vi "DSF.Engine.Timing.Max Concurrent Activations.vi"(8 "error in (no error)":errorcluster, 11 "Timings in":refnum<class "DSF.Engine.Timing.lvclass">[](array[class])) -> (0 "error out":errorcluster, 3 "Timings out":refnum<class "DSF.Engine.Timing.lvclass">[](array[class]))   [LabVIEW 2017, in "DSF.Engine.lvlib" / "DSF.Engine.Timing.lvclass"]
uses:
  DSF.Engine.Timing.lvclass
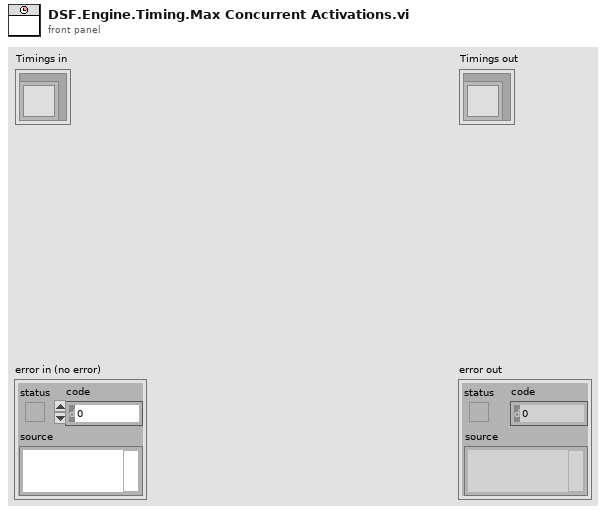
[diagram p1: front panel]
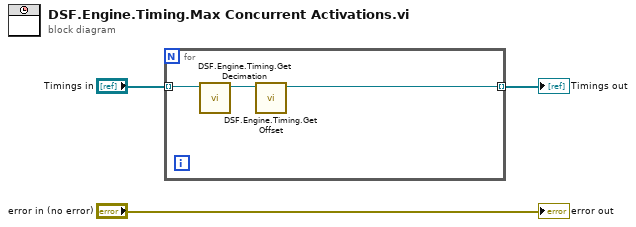
[diagram p0: block diagram]
diagram:
  n1 = for {
    tunnel: "Timings in" -> [w6] mode=indexing
    tunnel: [w4] -> w1 mode=indexing
    n2 = call "DSF.Engine.Timing.Get Decimation.vi"("Timing in"=w6) -> ("Timing out"=w5:refnum<class "DSF.Engine.Timing.lvclass">)  [unwired: 9 in, 1 out]
    n3 = call "DSF.Engine.Timing.Get Offset.vi"("Timing in"=w5) -> ("Timing out"=w4:refnum<class "DSF.Engine.Timing.lvclass">)  [unwired: 9 in, 1 out]
  }
  "Timings out" <- w1
  "error out" <- "error in (no error)"
